vi "DirettoreStatus.vi"(0 "FPGAReference":refnum<k20>) -> (4 "Counter":i32)   [LabVIEW 2012]
uses:
  <vilib>/Utility/error.llb/Error Cluster From Error Code.vi
  <vilib>/rvi/errors/niLvFpgaAdjustHostInterfaceError.vi
  <vilib>/rvi/interface/nirviMethod/nirviMethod.xnode
  <vilib>/FPGAPlugInAG/Dynamic/niLvFpga_ReadFifo_Dynamic.vi
  <vilib>/rvi/errors/niLvFpgaMergeErrorWithErrorCode.vi
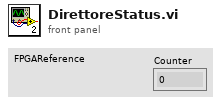
[diagram p1: front panel]
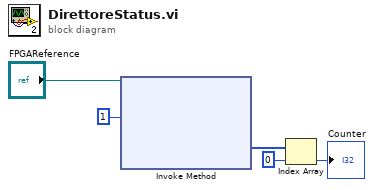
[diagram p0: block diagram]
diagram:
  n1 = xnode "Invoke Method"("FPGA VI Reference In"="FPGAReference", "Number of Elements"=u32 1) -> ("Data"=w3:i32[])  [unwired: 2 in, 3 out]
  n2 = Index Array(array=w3, index=0) -> (element=→"Counter":i32)
